vi "SignalReference.vi"(0 "Offset":dbl, 5 "Frequence 2":dbl, 7 "waveform en sortie":waveform(dbl), 9 "Amplitude":dbl, 11 "Signal de Reference":T1(ring), 12 "Phase":dbl) -> (15 "Tableau":waveform(dbl)[](array[waveform]))   [LabVIEW 2013]
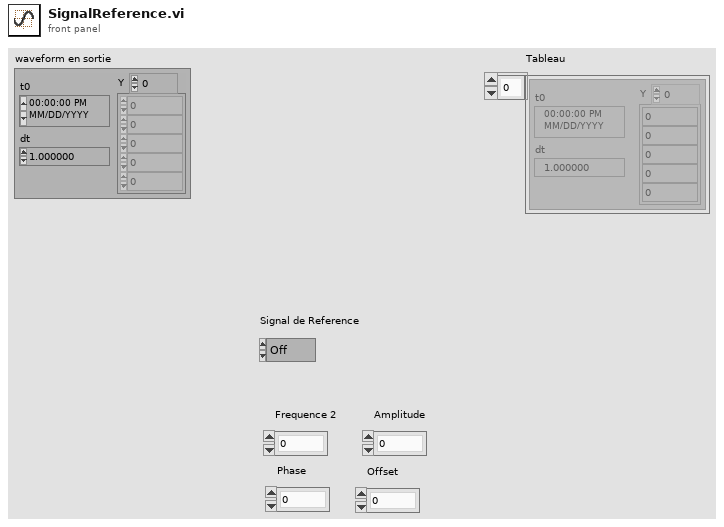
[diagram p1: front panel]
types:
  T1 = enum16{"Off", "Sinus", "Carre", "Triangle", "Scie"}
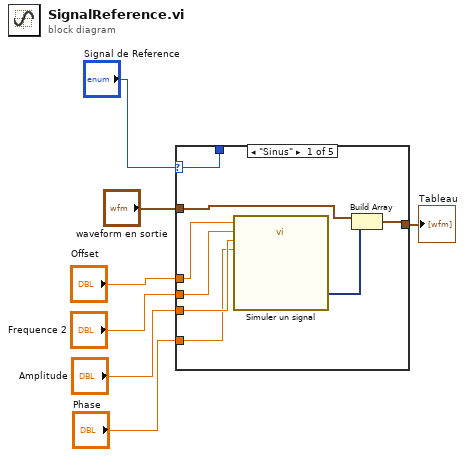
[diagram p0: block diagram]
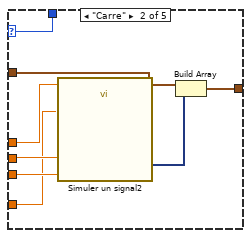
[diagram p2: hidden frame]
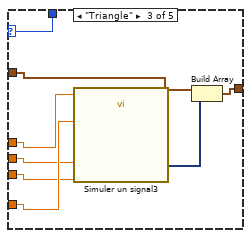
[diagram p3: hidden frame]
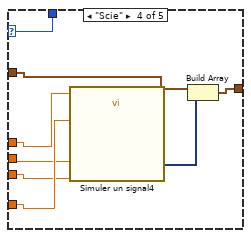
[diagram p4: hidden frame]
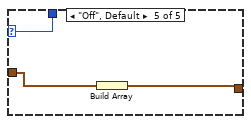
[diagram p5: hidden frame]
diagram:
  n1 = case shown="\"Sinus\"" "Signal de Reference" {
    selector: "Signal de Reference" -> [w8 w16 w24 w32 w40]
    tunnel: "Offset" -> [w13 w23 w27 w35 _]
    tunnel: "Frequence 2" -> [w12 w22 w28 w36 _]
    tunnel: "Amplitude" -> [w11 w21 w29 w37 _]
    tunnel: "Phase" -> [w10 w20 w30 w38 _]
    tunnel: "waveform en sortie" -> [w9 w18 w26 w34 w42]
    tunnel: [w14 w17 w25 w33 w41] -> w2
    tunnel: [w8 w16 w24 w32 w40] -> _
    frame "Sinus" {
      n2 = call "Simuler un signal"("Offset"=w13, "Frequency"=w12, "Amplitude"=w11, "Phase"=w10) -> ("Sinus"=w15:dynamicdata)  [unwired: 10 in, 1 out]
      n3 = Build Array(w9, w15) -> (w14:waveform(dbl)[])
    }
    frame "Carre" {
      n4 = call "Simuler un signal2"("Offset"=w23, "Frequency"=w22, "Amplitude"=w21, "Phase"=w20) -> ("Carré"=w19:dynamicdata)  [unwired: 10 in, 1 out]
      n5 = Build Array(w18, w19) -> (w17:waveform(dbl)[])
    }
    frame "Triangle" {
      n6 = call "Simuler un signal3"("Offset"=w27, "Frequency"=w28, "Amplitude"=w29, "Phase"=w30) -> ("Triangle"=w31:dynamicdata)  [unwired: 10 in, 1 out]
      n7 = Build Array(w26, w31) -> (w25:waveform(dbl)[])
    }
    frame "Scie" {
      n8 = call "Simuler un signal4"("Offset"=w35, "Frequency"=w36, "Amplitude"=w37, "Phase"=w38) -> ("Dents de scie"=w39:dynamicdata)  [unwired: 10 in, 1 out]
      n9 = Build Array(w34, w39) -> (w33:waveform(dbl)[])
    }
    frame "Off", Default {
      n10 = Build Array(w42) -> (w41:waveform(dbl)[])
    }
  }
  "Tableau" <- w2
